vi "Close.vi"(8 "error in (no error)":errorcluster, 11 "UDP in":refnum<class "UDP.lvclass">) -> (0 "error out":errorcluster, 3 "UDP out":refnum<class "UDP.lvclass">)   [LabVIEW 2019, in "Protocols.lvlib" / "UDP.lvclass"]
uses:
  UDP.lvclass
  UDP.lvclass/UDP.ctl
  Data Access/Read UDP Ref.vi
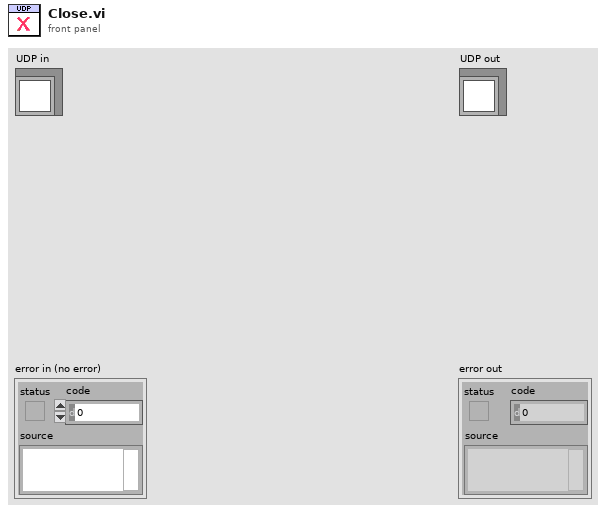
[diagram p1: front panel]
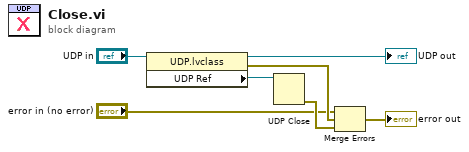
[diagram p0: block diagram]
diagram:
  n1 = property class="UDP.lvclass"(reference="UDP in") -> (reference out=→"UDP out":refnum<class "UDP.lvclass">, error out=w5:errorcluster, "UDP Ref"=w7:refnum<k16>)  [unwired: 1 in]
  n2 = UDP Close(connection ID=w7) -> (error out=w6:errorcluster)  [unwired: 1 in, 1 out]
  n3 = Merge Errors("error in (no error)", w5, w6) -> (→"error out":errorcluster)
